vi "svx_Polar_TreeInitialize.vi"(7 "XControl Name":string="Polar Plot", 10 "Display State In":T1={"Property Name"=[], "Container bounds"={"Width"=550, "Height"=250}, "Scale range"={"Maximum"=1.0, "Increment"=1.0}, "PointIdx"=0, "Marker list"=[], "Color settings"={"Arrow color"=16860, "Magnitude major grid"=13816530, "Magnitude minor grid"=16777216, "Phase grid"=13816530, "Phase scale marker text"=0}, "Magnitude scale name"="Magnitude", "Magnitude scale format string"="%#.2e", "MagnitudeScale:Visible"=TRUE, "MagnitudeScaleLabel:Visible"=TRUE, "PhaseScale:Visible"=TRUE, "Marker:Visible"=TRUE, "Cursor:Visible"=FALSE, "CursorName:Visible"=TRUE, "Autoscale"=TRUE, "Marker color"=16860, "Line color"=16711680, "Cursor color"=16711680, "Magnitude scale marker color"=0, "Plot.Line Style"=0, "Plot.Line Width"=0, "Plot.Point Style"=0, "Cursor.Line Style"=0, "Cursor.Line Width"=0, "Cursor.Point Style"=0, "Cursor.Style"=4, "Marker.Point Style"=2, "Point/fill color"=16711680, "Background color"=16777225, "Cursor name"="", "Cursor Release"=refnum, "Scale Range Change"=refnum, "data size(s)"=[], "Selectors:Visible"=TRUE, "Selector:ring Strings"={"Selector:Custom Strings"=FALSE, "Selector:Row Strings []"=[], "Selector:Column Strings []"=[], "User:Row Strings []"=[], "User:Column Strings []"=[]}, "Lock Cursor Info Position"=FALSE, "CursLoc"={"magnitude"=0.0, "phase"=0.0, "time/rev/RPM"=0.0}, "Plot Area:Position"={"Left"=0, "Top"=0}, "Plot Area:Size"={"Width"=0, "Height"=0}, "Marker.Style"=0, "Indication Arcs"=[], "Arc.Selector"=0, "customized marker"=[], "tree Width"=0, " Parents Tags"=[], "Children Tags"=[], "open?"=[], "index"=[{"row index"=0, "column index"=0}], "Label"="", "custom strings changed"=FALSE, "Owning VI"=refnum, "Legend BG color"=16777225, "Legend font color"=0, "column Width"=203, "attribute"=variant} caption="State", 11 "Tree ref in":refnum<vi>) -> (0 "All Children Tags":string[](array[string]), 1 "All Parents Tags":string[](array[string]), 2 "Display State out":T1={"Property Name"=[], "Container bounds"={"Width"=550, "Height"=250}, "Scale range"={"Maximum"=1.0, "Increment"=1.0}, "PointIdx"=0, "Marker list"=[], "Color settings"={"Arrow color"=16860, "Magnitude major grid"=13816530, "Magnitude minor grid"=16777216, "Phase grid"=13816530, "Phase scale marker text"=0}, "Magnitude scale name"="Magnitude", "Magnitude scale format string"="%#.2e", "MagnitudeScale:Visible"=TRUE, "MagnitudeScaleLabel:Visible"=TRUE, "PhaseScale:Visible"=TRUE, "Marker:Visible"=TRUE, "Cursor:Visible"=FALSE, "CursorName:Visible"=TRUE, "Autoscale"=TRUE, "Marker color"=16860, "Line color"=16711680, "Cursor color"=16711680, "Magnitude scale marker color"=0, "Plot.Line Style"=0, "Plot.Line Width"=0, "Plot.Point Style"=0, "Cursor.Line Style"=0, "Cursor.Line Width"=0, "Cursor.Point Style"=0, "Cursor.Style"=4, "Marker.Point Style"=2, "Point/fill color"=16711680, "Background color"=16777225, "Cursor name"="", "Cursor Release"=refnum, "Scale Range Change"=refnum, "data size(s)"=[], "Selectors:Visible"=TRUE, "Selector:ring Strings"={"Selector:Custom Strings"=FALSE, "Selector:Row Strings []"=[], "Selector:Column Strings []"=[], "User:Row Strings []"=[], "User:Column Strings []"=[]}, "Lock Cursor Info Position"=FALSE, "CursLoc"={"magnitude"=0.0, "phase"=0.0, "time/rev/RPM"=0.0}, "Plot Area:Position"={"Left"=0, "Top"=0}, "Plot Area:Size"={"Width"=0, "Height"=0}, "Marker.Style"=0, "Indication Arcs"=[], "Arc.Selector"=0, "customized marker"=[], "tree Width"=0, " Parents Tags"=[], "Children Tags"=[], "open?"=[], "index"=[{"row index"=0, "column index"=0}], "Label"="", "custom strings changed"=FALSE, "Owning VI"=refnum, "Legend BG color"=16777225, "Legend font color"=0, "column Width"=203, "attribute"=variant} caption="State", 3 "Tree ref out":refnum<vi>)   [LabVIEW 2017, in "SVX Polar Plot.xctl"]
uses:
  <vilib>/addons/_XControls/Polar Plot/SVX Polar Plot.xctl
  <vilib>/addons/_XControls/Polar Plot/subVIs/svx_Polar_Plot_Internal_State.ctl
  <vilib>/addons/_XControls/Polar Plot/subVIs/svx_Polar_Indication_Arcs.ctl
  <vilib>/addons/_XControls/Polar Plot/subVIs/svx_Polar_Customized_Markers.ctl
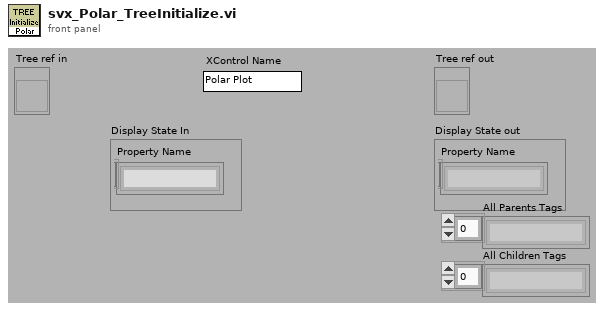
[diagram p1: front panel]
types:
  T1 = typedef "SVX Polar Plot.xctl/svx_Polar_Plot_Internal_State.ctl" = cluster{"Property Name":string[], "Container bounds":cluster{"Width":u32, "Height":u32}, "Scale range":cluster{"Maximum":dbl, "Increment":dbl}, "PointIdx":i32, "Marker list":cluster{"Name":string, "Color":u32, "Style":u8, "Point Style":u8, "Name Visible":bool, "Allow Drag":bool, "Annotation Mode":u32, "Plot":i32, "Index":i32, "Position":cluster{"X":dbl, "Y":dbl}, "X Scale":u32, "Y Scale":u32, "Show Arrow":bool, "Lock Name":bool, "Plot Area":i32, "Label Offset":cluster{"X":dbl, "Y":dbl}}[], "Color settings":cluster{"Arrow color":u32, "Magnitude major grid":u32, "Magnitude minor grid":u32, "Phase grid":u32, "Phase scale marker text":u32}, "Magnitude scale name":string, "Magnitude scale format string":string, "MagnitudeScale:Visible":bool, "MagnitudeScaleLabel:Visible":bool, "PhaseScale:Visible":bool, "Marker:Visible":bool, "Cursor:Visible":bool, "CursorName:Visible":bool, "Autoscale":bool, "Marker color":u32, "Line color":u32, "Cursor color":u32, "Magnitude scale marker color":u32, "Plot.Line Style":i32, "Plot.Line Width":i32, "Plot.Point Style":i32, "Cursor.Line Style":i32, "Cursor.Line Width":i32, "Cursor.Point Style":i32, "Cursor.Style":i32, "Marker.Point Style":i32, "Point/fill color":u32, "Background color":u32, "Cursor name":string, "Cursor Release":refnum<user-event>, "Scale Range Change":refnum<user-event>, "data size(s)":i32[], "Selectors:Visible":bool, "Selector:ring Strings":cluster{"Selector:Custom Strings":bool, "Selector:Row Strings []":string[], "Selector:Column Strings []":string[], "User:Row Strings []":string[], "User:Column Strings []":string[]}, "Lock Cursor Info Position":bool, "CursLoc":cluster{"magnitude":dbl, "phase":dbl, "time/rev/RPM":dbl}, "Plot Area:Position":cluster{"Left":i32, "Top":i32}, "Plot Area:Size":cluster{"Width":u32, "Height":u32}, "Marker.Style":i32, "Indication Arcs":T2, "Arc.Selector":u16, "customized marker":T3, "tree Width":u32, " Parents Tags":string[], "Children Tags":string[], "open?":bool[], "index":cluster{"row index":i32, "column index":i32}[], "Label":string, "custom strings changed":bool, "Owning VI":refnum<vi>, "Legend BG color":u32, "Legend font color":u32, "column Width":u32, "attribute":variant}
  T2 = typedef "SVX Polar Plot.xctl/svx_Polar_Indication_Arcs.ctl" = cluster{"Name":string, "Start radius":dbl, "End radius":dbl, "Line Style":i32, "Line Width":i32, "Border color":u32, "Fill color":u32, "Start angle":i16, "End angle":i16, "Visible":bool}[]
  T3 = typedef "SVX Polar Plot.xctl/svx_Polar_Customized_Markers.ctl" = cluster{"Name":string, "Color":u32, "Style":u8, "Point Style":u8, "Name Visible":bool, "Allow Drag":bool, "Annotation Mode":u32, "Plot":i32, "Index":i32, "Position":cluster{"Magnitude":dbl, "Phase":dbl}, "X Scale":u32, "Y Scale":u32, "Show Arrow":bool, "Lock Name":bool, "Plot Area":i32, "Label Offset":cluster{"Magnitude":dbl, "Phase":dbl}}[]
  T4 = enum16{"User-specified Font", "Application Font", "System Font", "Dialog Font"}
  T5 = cluster{"Left Cell String":string, "Child Text":string[], "Child Tag":string, "Item Indent":i32, "Child Only?":bool, "Glyph Index":i32}
  T6 = cluster{"Left Cell String":string, "Child Text":string[], "Child Tag":string, "Item Indent":i32, "Child Only?":bool, "Glyph Index":i32}[]
  T7 = cluster{"left":i16, "top":i16, "right":i16, "bottom":i16}
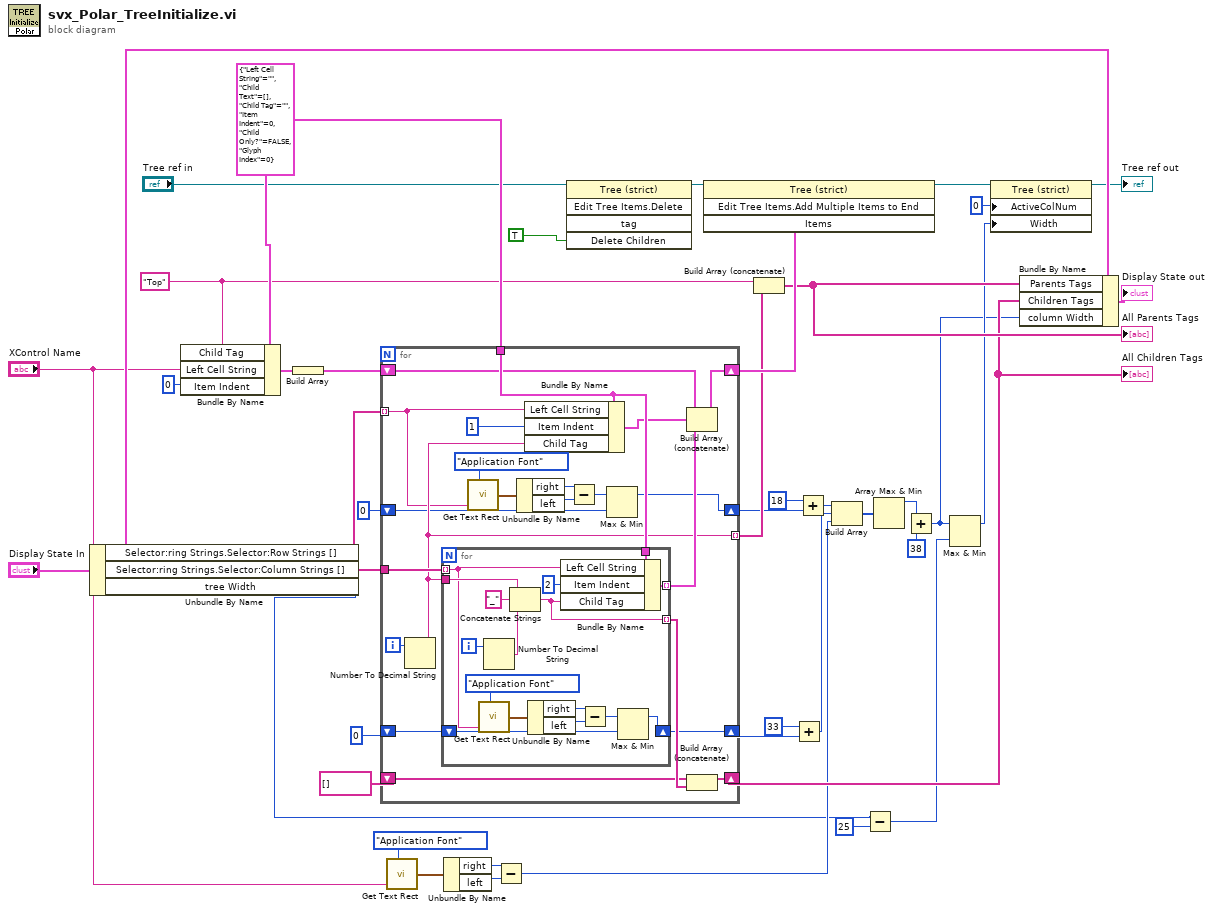
[diagram p0: block diagram]
diagram:
  w33 = "Top" ("Child Tag")
  w41 = T5 {"Left Cell String"="", "Child Text"=[], "Child Tag"="", "Item Indent"=0, "Child Only?"=FALSE, "Glyph Index"=0} ("element")
  n1 = Unbundle By Name("Display State In") -> ("Selector:ring Strings.Selector:Row Strings []"=w31:string[], "Selector:ring Strings.Selector:Column Strings []"=w30:string[], "tree Width"=w5:u32)
  n2 = Bundle By Name(cluster=w41, "Child Tag"=w33, "Left Cell String"="XControl Name", "Item Indent"=0) -> (w40:T5)
  n3 = Build Array(w40) -> (w39:T6)
  n4 = for {
    tunnel: w41 -> [w63]
    tunnel: w31 -> [w46] mode=indexing
    shift-right: [w59] -> w36
    shift-left: w39 -> [w60]
    tunnel: w30 -> [w64]
    shift-right: [w54] -> w26
    shift-left: string[] [] -> [w55]
    tunnel: [w53] -> w32 mode=indexing
    shift-right: [w45] -> w18
    shift-left: i16 0 ("x-y") -> [w47]
    shift-right: [w43] -> w15
    shift-left: i16 0 ("x-y") -> [w44]
    i -> [w57]
    n5 = Number To Decimal String(number=w57) -> (decimal integer string=w53:string)  [unwired: 1 in]
    n6 = for {
      tunnel: w64 -> [w65] mode=indexing
      tunnel: w63 -> [w80]
      tunnel: [w78] -> w58 mode=indexing
      tunnel: [w76] -> w56 mode=indexing
      tunnel: w53 -> [w75]
      shift-right: [w66] -> w43
      shift-left: w44 -> [w67]
      i -> [w74]
      n7 = call <vilib>:"Get Text Rect.vi"("desired font(Application)"=T4."Application Font", "text"=w65) -> ("rect"=w70:T7)  [unwired: 7 in]
      n8 = Number To Decimal String(number=w74) -> (decimal integer string=w73:string)  [unwired: 1 in]
      n9 = Concatenate Strings(w75, "_" ("string"), w73) -> (w76:string)
      n10 = Unbundle By Name(w70) -> ("right"=w71:i16, "left"=w72:i16)
      n11 = Bundle By Name(cluster=w80, "Left Cell String"=w65, "Item Indent"=2, "Child Tag"=w76) -> (w78:T5)
      n12 = Subtract(x=w71, y=w72) -> (x-y=w68:i16)
      n13 = Max & Min(x=w68, y=w67) -> (max(x,y)=w66:i16)  [unwired: 1 out]
    }
    n14 = call <vilib>:"Get Text Rect.vi"("desired font(Application)"=T4."Application Font", "text"=w46) -> ("rect"=w50:T7)  [unwired: 7 in]
    n15 = Unbundle By Name(w50) -> ("right"=w49:i16, "left"=w48:i16)
    n16 = Bundle By Name(cluster=w63, "Left Cell String"=w46, "Item Indent"=1, "Child Tag"=w53) -> (w61:T5)
    n17 = Subtract(x=w49, y=w48) -> (x-y=w52:i16)
    n18 = Max & Min(x=w52, y=w47) -> (max(x,y)=w45:i16)  [unwired: 1 out]
    n19 = Build Array (concatenate)(w60, w61, w58) -> (w59:T6)
    n20 = Build Array (concatenate)(w55, w56) -> (w54:string[])
  }
  "All Children Tags" <- w26
  n21 = call <vilib>:"Get Text Rect.vi"("desired font(Application)"=T4."Application Font", "text"="XControl Name") -> ("rect"=w23:T7)  [unwired: 7 in]
  n22 = Unbundle By Name(w23) -> ("right"=w24:i16, "left"=w25:i16)
  n23 = Subtract(x=w24, y=w25) -> (x-y=w12:i16)
  n24 = invoke on="Invoke Node" class="Tree (strict)" method="Edit Tree Items.Delete"(reference="Tree ref in", "Delete Children"=TRUE ("Delete Children?")) -> (reference out=w37:refnum<vi>)  [unwired: 3 in, 4 out]
  n25 = invoke on="Invoke Node" class="Tree (strict)" method="Edit Tree Items.Add Multiple Items to End"(reference=w37, "Items"=w36) -> (reference out=w8:refnum<vi>)  [unwired: 2 in, 3 out]
  n26 = Build Array (concatenate)(w33, w32) -> (w27:string[])
  "All Parents Tags" <- w27
  n27 = Add(x=i16 33, y=w15) -> (x+y=w13:i16)
  n28 = Add(x=i16 18, y=w18) -> (x+y=w14:i16)
  n29 = Build Array(w14, w13, w12) -> (w9:i16[])
  n30 = Subtract(x=w5, y=u32 25) -> (x-y=w3:u32)
  n31 = Array Max & Min(array=w9) -> (max value=w10:i16)  [unwired: 3 out]
  n32 = Add(x=w10, y=i16 38) -> (x+y=w1:i16)
  n33 = Max & Min(x=w1, y=w3) -> (max(x,y)=w2:u32)  [unwired: 1 out]
  n34 = property class="Tree (strict)"(reference=w8, "ActiveColNum"=0 ("Active Cell:Active Column Number"), "Width"=w2) -> (reference out=→"Tree ref out":refnum<vi>)  [unwired: 1 in, 1 out]
  n35 = Bundle By Name(cluster="Display State In", "Parents Tags"=w27, "Children Tags"=w26, "column Width"=w1) -> (→"Display State out":T1)
